vi "Display FI locations on tiled image.vi"(5 "[user-specified font]":T1={"Font Name:"="", "Size"=8, "Strikeout?"=FALSE, "Italic?"=FALSE, "Underline?"=FALSE, "Outline?"=FALSE, "Shadow?"=FALSE, "Bold?"=FALSE}, 6 "Symbol":string="+", 7 "Primary grid @ green":bool=TRUE, 8 "Tiled Image fit to":u8(ring) items=["Width", "Height"], 9 "Focus Index Options":T2={"Keep aspect ratio"=FALSE, "Show Focus Index"=TRUE, "Focus Index primary grid center"=TRUE, "X Grids"=[[1]], "Y Grids"=[[1]], "Primary X index"=[[1]], "Primary Y index"=[[1]]} {"Y Grids" step=2; "X Grids" step=2}, 10 "SEM Scan Parameters":T3={"X size (um)"=80.0, "Y size (um)"=80.0, "X center (um)"=0.0, "Y center (um)"=0.0, "X size (V)"=3.7333333333333334, "X size auto"=TRUE, "X stig"=[[0.0]], "Y stig"=[[0.0]], "X aln"=[[0.0]], "Y aln"=[[0.0]], "Scan rate (Hz)"=10000000, "Oversampling"=5, "Oversampling auto"=TRUE, "Frame line rampdown ratio"=0.1, "Pixel size (nm)"=8.0, "WD (mm)"=[[3.0]], "X tiles"=1, "Y tiles"=1, "Overlap (um)"=2.0, "Interlaced"=TRUE, "dX (um)"=[0.0], "dY (um)"=[0.0], "Frames"=1} {"dY (um)" format="%.1f"; "dX (um)" format="%.1f"; "Frames" min=1 step=1; "WD (mm)" step=0.001 format="%.4f"; "Y aln" format="%.1f"; "X aln" format="%.1f"; "Y stig" format="%.1f"; "X stig" format="%.1f"; "Overlap (um)" min=0; "Y tiles" min=1; "X tiles" min=1; "X size (um)" format="%.2f"; "Y size (um)" format="%.2f"; "Frame line rampdown ratio" min=0 max=1 step=0.05 format="%.2g"; "X center (um)" step=1 format="%.3f"; "Y center (um)" step=1 format="%.3f"; "X size (V)" format="%_4g"; "Scan rate (Hz)" max=4000000 step=100000 format="%.2e"}, 11 "Image reference":refnum<vi>) -> ()   [LabVIEW 2018]
panel:
  # "Grids"
  # "Primary"
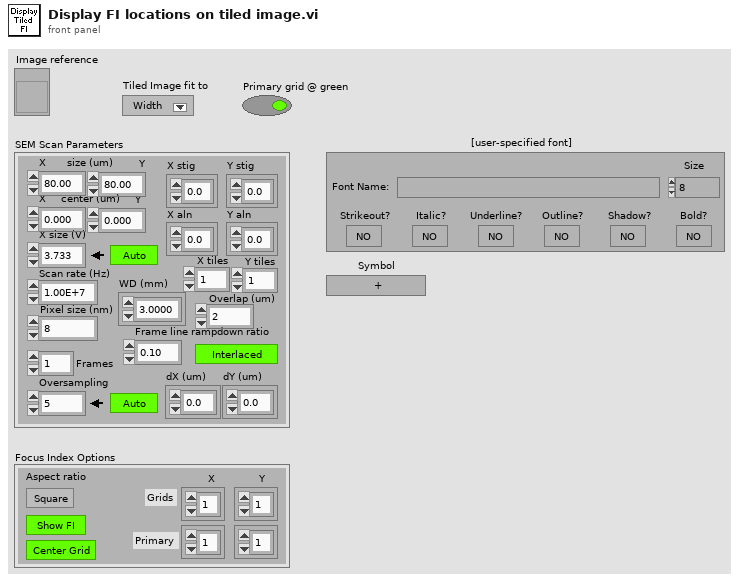
[diagram p1: front panel]
types:
  T1 = cluster{"Font Name:":string, "Size":i16, "Strikeout?":bool, "Italic?":bool, "Underline?":bool, "Outline?":bool, "Shadow?":bool, "Bold?":bool}
  T2 = cluster{"Keep aspect ratio":bool, "Show Focus Index":bool, "Focus Index primary grid center":bool, "X Grids":u8[][], "Y Grids":u8[][], "Primary X index":u8[][], "Primary Y index":u8[][]}
  T3 = cluster{"X size (um)":sgl, "Y size (um)":sgl, "X center (um)":sgl, "Y center (um)":sgl, "X size (V)":dbl, "X size auto":bool, "X stig":sgl[][], "Y stig":sgl[][], "X aln":sgl[][], "Y aln":sgl[][], "Scan rate (Hz)":u32, "Oversampling":u32, "Oversampling auto":bool, "Frame line rampdown ratio":sgl, "Pixel size (nm)":sgl, "WD (mm)":sgl[][], "X tiles":u8, "Y tiles":u8, "Overlap (um)":sgl, "Interlaced":bool, "dX (um)":sgl[], "dY (um)":sgl[], "Frames":u8}
  T4 = cluster{"horizontal":enum16{"left", "center", "right"}, "vertical":enum16{"top", "center", "bottom"}}
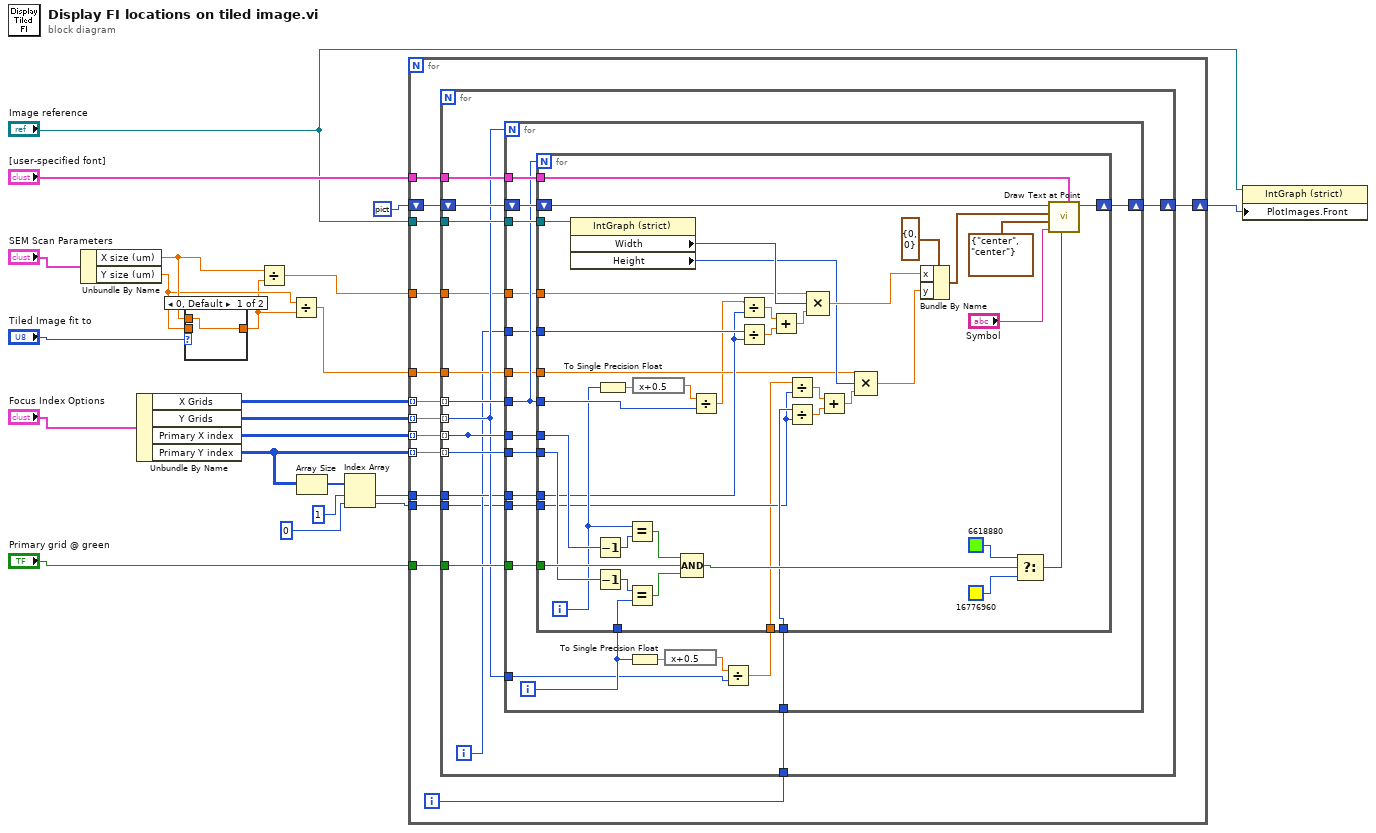
[diagram p0: block diagram]
diagram:
  n1 = Unbundle By Name("SEM Scan Parameters") -> ("X size (um)"=w13:sgl, "Y size (um)"=w12:sgl)
  n2 = Unbundle By Name("Focus Index Options") -> ("X Grids"=w20:u8[][], "Y Grids"=w19:u8[][], "Primary X index"=w17:u8[][], "Primary Y index"=w5:u8[][])
  n3 = case shown="0, Default" "Tiled Image fit to" {
    tunnel: w13 -> [w23 _]
    tunnel: w12 -> [_ w24]
    tunnel: [w23 w24] -> w11
    frame 0, Default {
    }
    frame 1 {
    }
  }
  n4 = Divide(x=w13, y=w11) -> (x/y=w10:sgl)
  n5 = Divide(x=w12, y=w11) -> (x/y=w9:sgl)
  n6 = Array Size(array=w5) -> (size(s)=w6:i32[])
  n7 = Index Array(array=w6, index #1=1 ("index"), index #2=0 ("index")) -> (element #1=w4:i32, element #2=w3:i32)
  n8 = for {
    tunnel: w20 -> [w38] mode=indexing
    tunnel: w19 -> [w37] mode=indexing
    tunnel: "Image reference" -> [w36]
    shift-right: [w35] -> w2
    shift-left: picture data[5B] ("picture") -> [w34]
    tunnel: w17 -> [w33] mode=indexing
    tunnel: w5 -> [w32] mode=indexing
    tunnel: "[user-specified font]" -> [w31]
    tunnel: "Primary grid @ green" -> [w30]
    tunnel: w10 -> [w29]
    tunnel: w9 -> [w28]
    tunnel: w4 -> [w27]
    tunnel: w3 -> [w26]
    i -> [w25]
    n9 = for {
      tunnel: w38 -> [w53] mode=indexing
      tunnel: w37 -> [w45] mode=indexing
      tunnel: w36 -> [w52]
      shift-right: [w51] -> w35
      shift-left: w34 -> [w50]
      tunnel: [w47] -> _ mode=indexing
      tunnel: w33 -> [w47] mode=indexing
      tunnel: w32 -> [w46] mode=indexing
      tunnel: w31 -> [w49]
      tunnel: w30 -> [w48]
      tunnel: w29 -> [w44]
      tunnel: w28 -> [w43]
      tunnel: w27 -> [w42]
      tunnel: w26 -> [w40]
      tunnel: w25 -> [w39]
      i -> [w41]
      n10 = for {
        N: w45 -> [_]
        tunnel: w53 -> [w61]
        tunnel: w52 -> [w72]
        shift-right: [w71] -> w51
        shift-left: w50 -> [w70]
        tunnel: w49 -> [w69]
        tunnel: w48 -> [w68]
        tunnel: w47 -> [w67]
        tunnel: w46 -> [w66]
        tunnel: w45 -> [w62]
        tunnel: w44 -> [w60]
        tunnel: w43 -> [w58]
        tunnel: w42 -> [w57]
        tunnel: w41 -> [w56]
        tunnel: w40 -> [w55]
        tunnel: w39 -> [w54]
        i -> [w63]
        n11 = To Single Precision Float(number=w63) -> (single precision float=w64:sgl)
        n12 = expression code="x+0.5"(w64) -> (w65:sgl)
        n13 = Divide(x=w65, y=w62) -> (x/y=w59:sgl)
        n14 = for {
          N: w61 -> [_]
          tunnel: w72 -> [w111]
          shift-right: [w110] -> w71
          shift-left: w70 -> [w109]
          tunnel: w69 -> [w108]
          tunnel: w63 -> [w98]
          tunnel: w68 -> [w97]
          tunnel: w67 -> [w96]
          tunnel: w66 -> [w95]
          tunnel: w61 -> [w92]
          tunnel: w60 -> [w73]
          tunnel: w59 -> [w76]
          tunnel: w58 -> [w75]
          tunnel: w57 -> [w88]
          tunnel: w56 -> [w89]
          tunnel: w55 -> [w78]
          tunnel: w54 -> [w79]
          i -> [w91]
          n15 = property on="Property Node" class="IntGraph (strict)"(reference=w111) -> ("Width"=w85:u32, "Height"=w80:u32)  [unwired: 1 in, 2 out]
          n16 = Decrement(x=w96) -> (x-1=w102:u8)
          n17 = Decrement(x=w95) -> (x-1=w103:u8)
          n18 = To Single Precision Float(number=w91) -> (single precision float=w94:sgl)
          n19 = Equal?(x=w91, y=w102) -> (x = y?=w101:bool)
          n20 = Equal?(x=w103, y=w98) -> (x = y?=w100:bool)
          n21 = expression code="x+0.5"(w94) -> (w93:sgl)
          n22 = Compound Arithmetic op=AND(w101, w97, w100) -> (w99:bool)
          n23 = Divide(x=w93, y=w92) -> (x/y=w74:sgl)
          n24 = Divide(x=w74, y=w88) -> (x/y=w90:sgl)
          n25 = Divide(x=w89, y=w88) -> (x/y=w87:dbl)
          n26 = Add(x=w90, y=w87) -> (x+y=w86:dbl)
          n27 = Divide(x=w76, y=w78) -> (x/y=w81:sgl)
          n28 = Divide(x=w79, y=w78) -> (x/y=w82:dbl)
          n29 = Compound Arithmetic op=MULTIPLY(w73, w85, w86) -> (w84:dbl)
          n30 = Add(x=w81, y=w82) -> (x+y=w83:dbl)
          n31 = Compound Arithmetic op=MULTIPLY(w75, w80, w83) -> (w77:dbl)
          n32 = Bundle By Name(cluster=cluster{"x":i16, "y":i16} {"x"=0, "y"=0} ("origin"), "x"=w84, "y"=w77) -> (w112:cluster{"x":i16, "y":i16})
          n33 = Select(t=u32 6618880 ("text color(black)"), s=w99, f=u32 16776960 ("text color(black)")) -> (s? t:f=w104:u32)
          n34 = call <vilib>:"Draw Text at Point.vi"("[user-specified font]"=w108, "text color(black)"=w104, "text"="Symbol", "alignment(left, top)"=T4 {"horizontal"=enum."center", "vertical"=enum."center"}, "origin"=w112, "picture"=w109) -> ("new picture"=w110:picture)  [unwired: 4 in, 1 out]
        }
      }
    }
  }
  n35 = property on="Property Node" class="IntGraph (strict)"(reference="Image reference", "PlotImages.Front"=w2) -> ()  [unwired: 1 in, 2 out]
